vi "Configure Analog Bus.vi"(6 "Include Channel (F: Exclude)":bool, 7 "Enable Analog Bus Display (F: Disable)":bool, 8 "error in (no error)":errorcluster, 9 "Analog Bus Label (\"\")":string, 10 "Channel List (0)":string="0", 11 "VISA resource name":refnum<visa-resource-name>) -> (0 "error out":errorcluster, 3 "VISA resource name out":refnum<visa-resource-name>)   [LabVIEW 2023, in "Keysight-DSQx3014T.lvlib"]
doc: "Configures the analog bus.\n\nNote: This VI is only applicable for 1000 X-Series."
uses:
  Keysight-DSQx3014T.lvlib
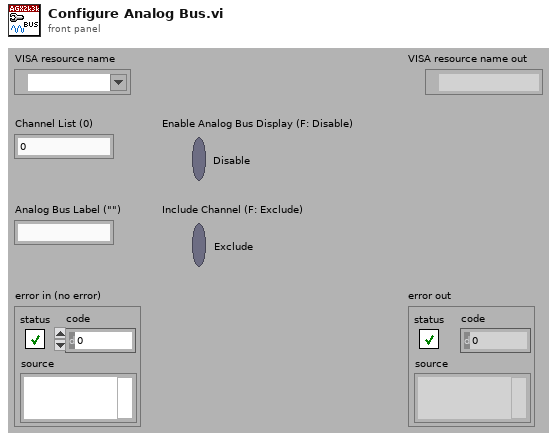
[diagram p1: front panel]
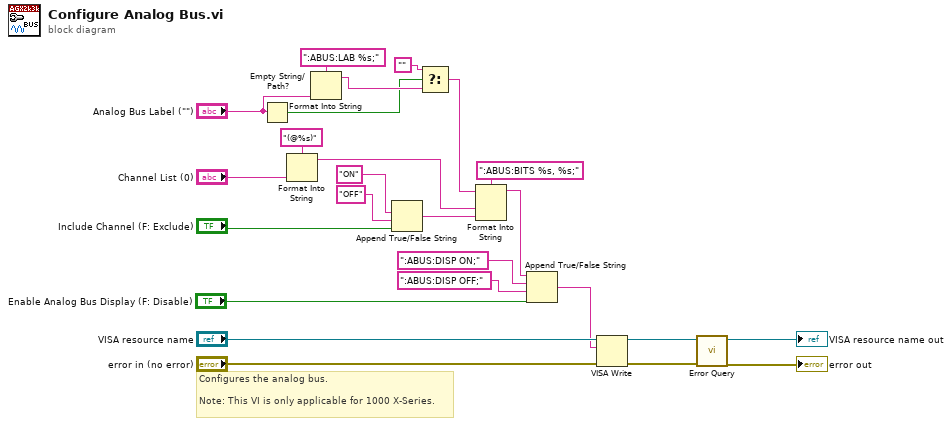
[diagram p0: block diagram]
diagram:
  # "Configures the analog bus.\n\nNote: This VI is only applicable for 1000 X-Series."
  n1 = Empty String/Path?(string/path="Analog Bus Label (\"\")") -> (empty?=w5:bool)
  n2 = Format Into String(format string="(@%s)", "Channel List (0)") -> (resulting string=w10:string)  [unwired: 2 in, 1 out]
  n3 = Format Into String(format string=":ABUS:LAB %s;", "Analog Bus Label (\"\")") -> (resulting string=w6:string)  [unwired: 2 in, 1 out]
  n4 = Append True/False String(1:"Include Channel (F: Exclude)", 2:"OFF", 3:"ON") -> (0:w17:string)  [unwired: 1 in]
  n5 = Select(t="", s=w5, f=w6) -> (s? t:f=w3:string)
  n6 = Format Into String(format string=":ABUS:BITS %s, %s;", initial string=w3, w10, w17) -> (resulting string=w2:string)  [unwired: 1 in, 1 out]
  n7 = Append True/False String(1:"Enable Analog Bus Display (F: Disable)", 2:":ABUS:DISP OFF;", 3:":ABUS:DISP ON;", 4:w2) -> (0:w1:string)
  n8 = VISA Write(VISA resource name="VISA resource name", write buffer=w1, error in (no error)="error in (no error)") -> (VISA resource name out=w14:refnum<visa-resource-name>, error out=w13:errorcluster)  [unwired: 1 out]
  n9 = call "Error Query.vi"("error in (no error)"=w13, "VISA resource name"=w14) -> ("error out"=→"error out":errorcluster, "VISA resource name out"=→"VISA resource name out":refnum<visa-resource-name>)  [unwired: 6 in, 2 out]
